vi "Create Cal File Array.vi"(1 "Cal Units":string[](array[string]), 2 "Cal Log OUT":string[][](array[string]), 3 "Available Channels":string[](array[string])) -> (0 "Cal Log OUT":string[][](array[string]))   [LabVIEW 2012]
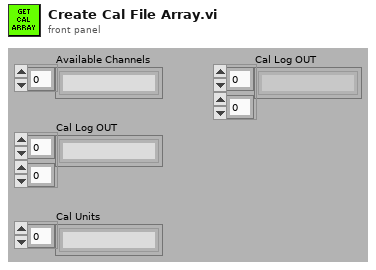
[diagram p1: front panel]
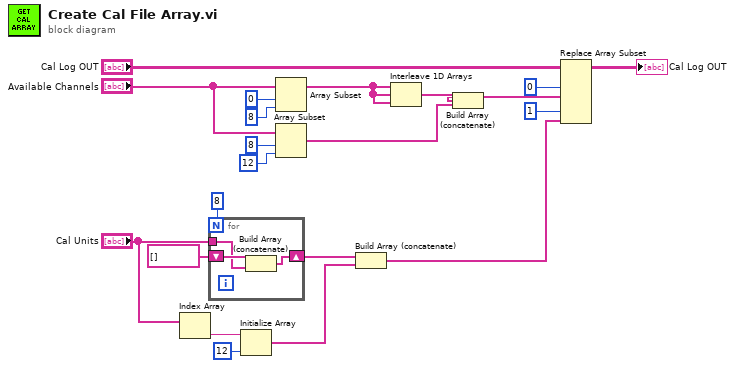
[diagram p0: block diagram]
diagram:
  n1 = Index Array(array="Cal Units") -> (element=w10:string)  [unwired: 1 in]
  n2 = for {
    N: 8 -> [_]
    tunnel: "Cal Units" -> [w22]
    shift-right: [w24] -> w12
    shift-left: string[] [] -> [w23]
    n3 = Build Array (concatenate)(w23, w22) -> (w24:string[])
  }
  n4 = Initialize Array(w10, 12 ("dimension size")) -> (w8:string[])
  n5 = Array Subset(array="Available Channels", index=0, length=8) -> (w13:string[])
  n6 = Array Subset(array="Available Channels", index=8, length=12) -> (w2:string[])
  n7 = Build Array (concatenate)(w12, w8) -> (w7:string[])
  n8 = Interleave 1D Arrays(w13, w13, w13) -> (w6:string[])
  n9 = Build Array (concatenate)(w6, w2) -> (w1:string[])
  n10 = Replace Array Subset(array="Cal Log OUT", new element #1=w1, index (col) #1=0 ("disabled index (col)"), new element #2=w7, index (col) #2=1 ("index (col)")) -> (→"Cal Log OUT":string[][])  [unwired: 2 in]
